vi "ep_Flicker Block2.vi"(0 "adapted voltage":dbl[](array[numeric])) -> (4 "squared voltage":dbl[](array[numeric]))   [LabVIEW 2011, in "NI_EP_Power Quality.lvlib"]
doc: "The purpose of this VI is to recover the voltage fluctuation by squaring the input voltage scaled to the reference level, thus simulating the behaviour of a lamp."
uses:
  <vilib>/addons/Electrical Power/PQ/NI_EP_Power Quality.lvlib
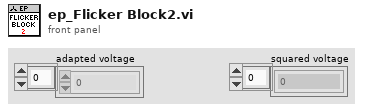
[diagram p1: front panel]
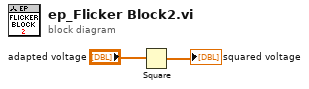
[diagram p0: block diagram]
diagram:
  n1 = Square(x="adapted voltage") -> (x^2=→"squared voltage":dbl[])
